vi "Run Filter.vi"(8 "error in (no error)":errorcluster, 10 "resource entries in":T1(array[cluster]) {"FPGA CD Ref" format="%.0x"; "reserver" format="%.0x"}, 11 "Filter in":refnum<class "Filter.lvclass">) -> (0 "error out":errorcluster, 2 "resource entries out":T1(array[cluster]) {"FPGA CD Ref" format="%.0x"; "reserver" format="%.0x"})   [LabVIEW 2016, in "FPGA Resource Manager.lvlib" / "Filter.lvclass"]
uses:
  FPGA RM Test Client Configuration.llb/Filter.lvclass
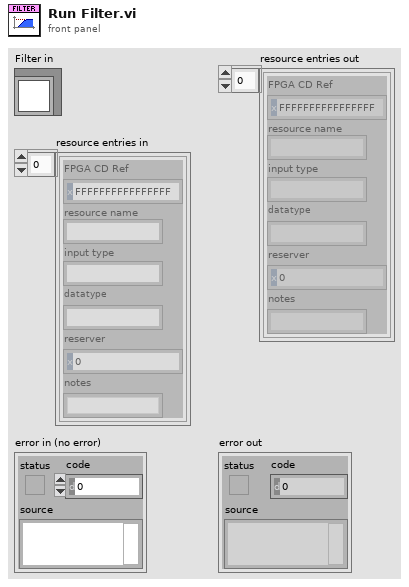
[diagram p1: front panel]
types:
  T1 = cluster{"FPGA CD Ref":u64, "resource name":string, "input type":string, "datatype":string, "reserver":u64, "notes":string}[]
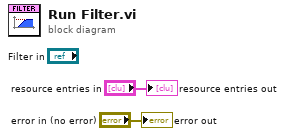
[diagram p0: block diagram]
diagram:
  "error out" <- "error in (no error)"
  "resource entries out" <- "resource entries in"
